vi "LeCroy data transfer.vi"() -> ()   [LabVIEW 2014]
uses:
  LV source/data.ctl
  <instrlib>/LeCroy Wave Series/LeCroy Wave Series.lvlib
panel:
  in  "OK Button":bool
  in  "file name":string="pulse"
  in  "Save to:":path=path "C:/Users/Andrii/Desktop/Data"
  in  "next index":dbl=12.0
  in  "Auto-indexing":bool=TRUE
  in  "Save to file":bool
  in  "Get waveforms":bool
  out "XY Graph":cluster{"Y":dbl[], "Y":dbl[]}(graph)
  out "Data from Source 2 (Y)":waveform(dbl)(graph)={"t0"=timestamp(0 s since 1904-01-01), "dt"=1.0000000116860974e-07, "Y"=array[100002 elements]}
  in  "Source 2 (Y)":u16(ring) items=["Channel 1", "Channel 2", "Channel 3", "Channel 4", "Memory 1", "Memory 2", "Memory 3", "Memory 4", "Function 1", "Function 2", "Function 3", "Function 4", "Function 5", "Function 6", "Function 7", "Function 8", "None"]
  in  "Source 1 (X)":u16(ring) items=["Channel 1", "Channel 2", "Channel 3", "Channel 4", "Memory 1", "Memory 2", "Memory 3", "Memory 4", "Function 1", "Function 2", "Function 3", "Function 4", "Function 5", "Function 6", "Function 7", "Function 8"]
  out "Data from Source 1 (X)":waveform(dbl)(graph)={"t0"=timestamp(0 s since 1904-01-01), "dt"=1.0000000116860974e-07, "Y"=array[100002 elements]}
  in  "VISA address of osciloscope":refnum<visa-resource-name>="USB0::0x05FF::0x1023::3106N58774::INSTR"
  # "Getting waveform from LeCroy\n\nConfigure the LeCroy scope manually and execute a SINGLE trigger to get a waveform on the desired channel."
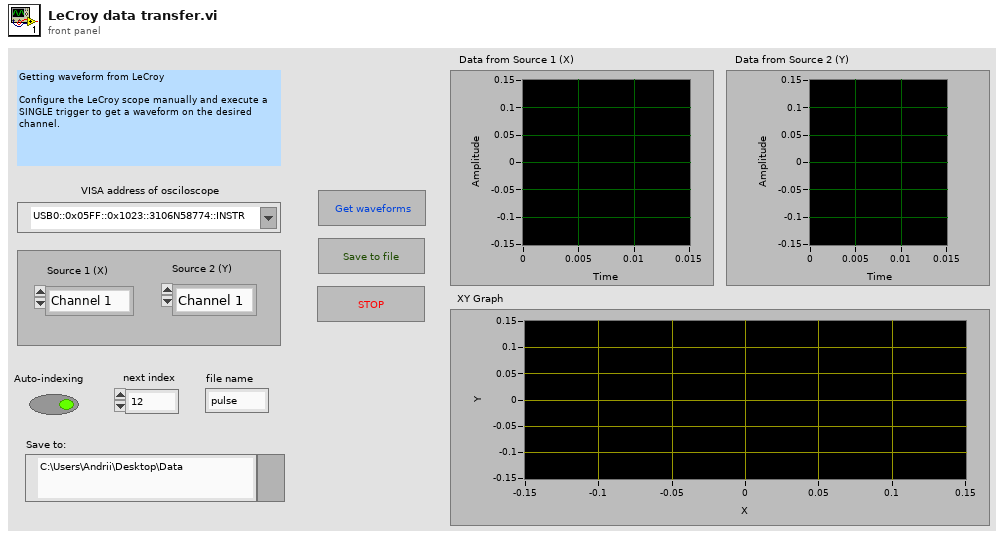
[diagram p1: front panel]
types:
  T1 = typedef "data.ctl" = cluster{"X-axis":dbl[], "Y-axis":dbl[], "time X":dbl[], "time Y":dbl[]}
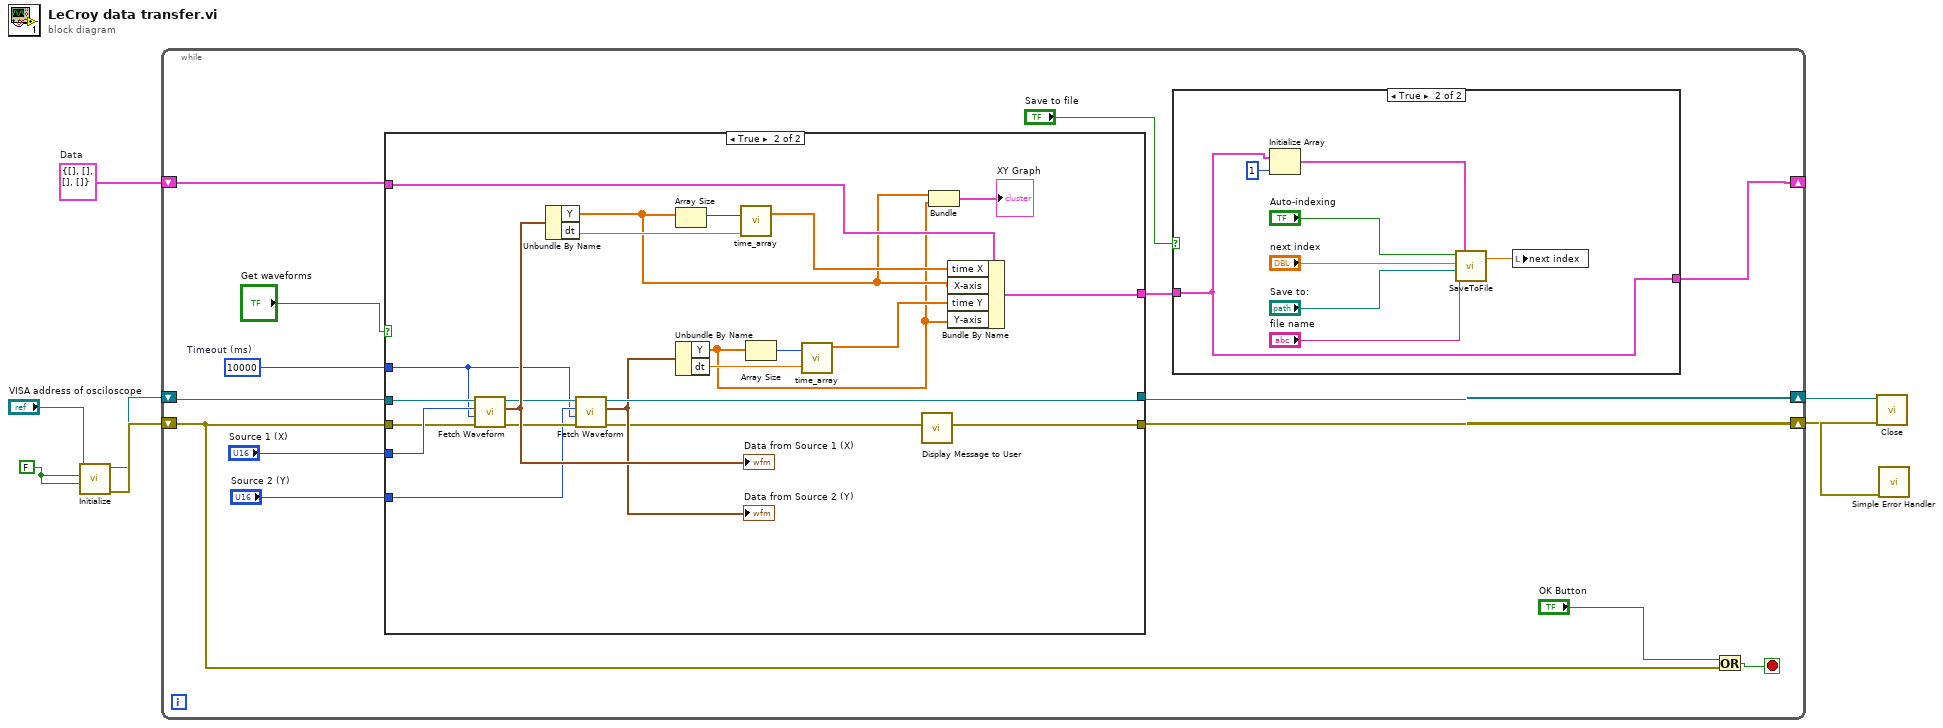
[diagram p0: block diagram]
diagram:
  w1 = T1 {"X-axis"=[], "Y-axis"=[], "time X"=[], "time Y"=[]}  # Data
  w4 = FALSE ("Reset? (T: Yes)")
  n1 = call "Initialize.vi"("Reset? (T: Yes)"=w4, "ID Query? (T: Yes)"=w4, "VISA resource name"="VISA address of osciloscope") -> ("error out"=w6:errorcluster, "VISA resource name out"=w5:refnum<visa-resource-name>)  [unwired: 7 in]
  n2 = while {
    shift-right: [w19] -> w2
    shift-left: w6 -> [w10]
    shift-right: [w20] -> w3
    shift-left: w5 -> [w21]
    shift-right: [w11] -> _
    shift-left: w1 -> [w12]
    stop <- w14 stop-if-true
    w17 = u32 10000  # Timeout (ms)
    n3 = case shown="True" "Get waveforms" {
      tunnel: "Source 1 (X)" -> [_ w57]
      tunnel: w10 -> [w34 w56]
      tunnel: w21 -> [w33 w55]
      tunnel: [w33 w51] -> w20
      tunnel: [w34 w35] -> w19
      tunnel: "Source 2 (Y)" -> [_ w50]
      tunnel: w17 -> [_ w49]
      tunnel: [w32 w47] -> w13
      tunnel: w12 -> [w32 w46]
      frame False {
      }
      frame True {
        n4 = call "Fetch Waveform.vi"("error in (no error)"=w56, "Timeout (10000 ms)"=w49, "Source (0: Channel 1)"=w57, "VISA resource name"=w55) -> ("error out"=w52:errorcluster, "Waveform Graph"=w54:waveform(dbl), "VISA resource name out"=w53:refnum<visa-resource-name>)  [unwired: 5 in]
        "Data from Source 1 (X)" <- w54
        n5 = Unbundle By Name(w54) -> ("Y"=w39:dbl[], "dt"=w44:dbl)
        n6 = call "Fetch Waveform.vi"("error in (no error)"=w52, "Timeout (10000 ms)"=w49, "Source (0: Channel 1)"=w50, "VISA resource name"=w53) -> ("error out"=w36:errorcluster, "Waveform Graph"=w48:waveform(dbl), "VISA resource name out"=w51:refnum<visa-resource-name>)  [unwired: 5 in]
        "Data from Source 2 (Y)" <- w48
        n7 = Array Size(array=w39) -> (size(s)=w43:i32)
        n8 = Unbundle By Name(w48) -> ("Y"=w37:dbl[], "dt"=w42:dbl)
        n9 = call "time_array.vi"("dt"=w44, "length"=w43) -> ("time"=w40:dbl[])  [unwired: 9 in]
        n10 = Array Size(array=w37) -> (size(s)=w41:i32)
        n11 = call "time_array.vi"("dt"=w42, "length"=w41) -> ("time"=w38:dbl[])  [unwired: 9 in]
        n12 = call "Display Message to User"("error in (no error)"=w36) -> ("error out"=w35:errorcluster)  [unwired: 9 in, 1 out]
        n13 = Bundle("Y"=w39, "Y"=w37) -> (→"XY Graph":cluster{"Y":dbl[], "Y":dbl[]})  [unwired: 1 in]
        n14 = Bundle By Name(cluster=w46, "time X"=w40, "X-axis"=w39, "time Y"=w38, "Y-axis"=w37) -> (w47:T1)
      }
    }
    n15 = case shown="True" "Save to file" {
      tunnel: w13 -> [w23 w24]
      tunnel: [w23 w24] -> w11
      frame False {
      }
      frame True {
        n16 = Initialize Array(w24, 1 ("dimension size")) -> (w26:T1[])
        n17 = call "SaveToFile.vi"("Autoindeksowanie"="Auto-indexing", "IndexIn"="next index", "Path"="Save to:", "next file"="file name", "Array"=w26) -> ("IndexOut"=w25:dbl)  [unwired: 1 in]
        n18 = local write "next index"(w25) -> ()
      }
    }
    n19 = Or(x="OK Button", y=w10) -> (x .or. y?=w14:bool)
  }
  n20 = call "Close.vi"("error in (no error)"=w2, "VISA resource name"=w3) -> ("error out"=w8:errorcluster)  [unwired: 9 in]
  n21 = call <vilib>:"Simple Error Handler.vi"("error in (no error)"=w8) -> ()  [unwired: 4 in, 5 out]
